vi "Configure Device.vi"(8 "error in":errorcluster, 11 "Vaisala Probe in":refnum<class "Vaisala.lvclass">) -> (0 "error out":errorcluster, 3 "Vaisala Probe out":refnum<class "Vaisala.lvclass">)   [LabVIEW 2015, in "Vaisala.lvclass"]
doc: "Configure the current instance of the Vaisala probe. In this case, we will get the correct address and then set the serial delayso that the probe responds in the correct amount of time. When configuration is done, make sure the session is closed."
uses:
  Vaisala.lvclass
  Instruments/Nicholas/Session/FPGA Serial Session.lvclass
  Reusable/Session APIs/File Access/Config Data/Config Data.lvclass
  Vaisala.lvclass/Vaisala.ctl
  Configurable Device/Configurable Device.lvclass/Configurable Device.ctl
  Reusable/Session APIs/File Access/Config Data/Config Data.lvclass/Config Data.ctl
  Reusable/Session APIs/Text Communication/Text Device Session.lvclass/Text Device Session.ctl
  Accessors/Read ID.vi
  Accessors/Read hSession.vi
  Configurable Device/Read Handle.vi
  Reusable/Session APIs/File Access/Config Data/Accessors/Read Ref.vi
  Reusable/Session APIs/Text Communication/Read hSysLog.vi
  <vilib>/Utility/config.llb/Read Key (I32).vi
  <userlib>/_Session Fwk/Session - Root.lvclass
  <vilib>/Utility/config.llb/NI_LVConfig.lvlib
  Reusable/Session APIs/Text Communication/Text Device Session.lvclass
  Reusable/Session APIs/Serial/Public/Get Data/Get String.vi
  Reusable/Session Log/System Log.lvclass
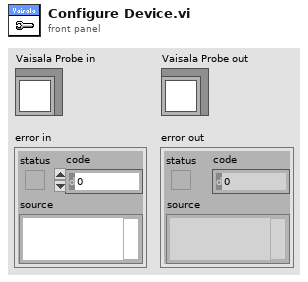
[diagram p1: front panel]
types:
  T1 = typedef "Session - Root.lvclass/Session Handle.ctl" = refnum<data-value>
  T2 = typedef "Config Data.lvclass/Config Session.ctl" = refnum<data-value>
  T3 = typedef "NI_LVConfig.lvlib/Config Data RefNum.ctl" = refnum<k1>
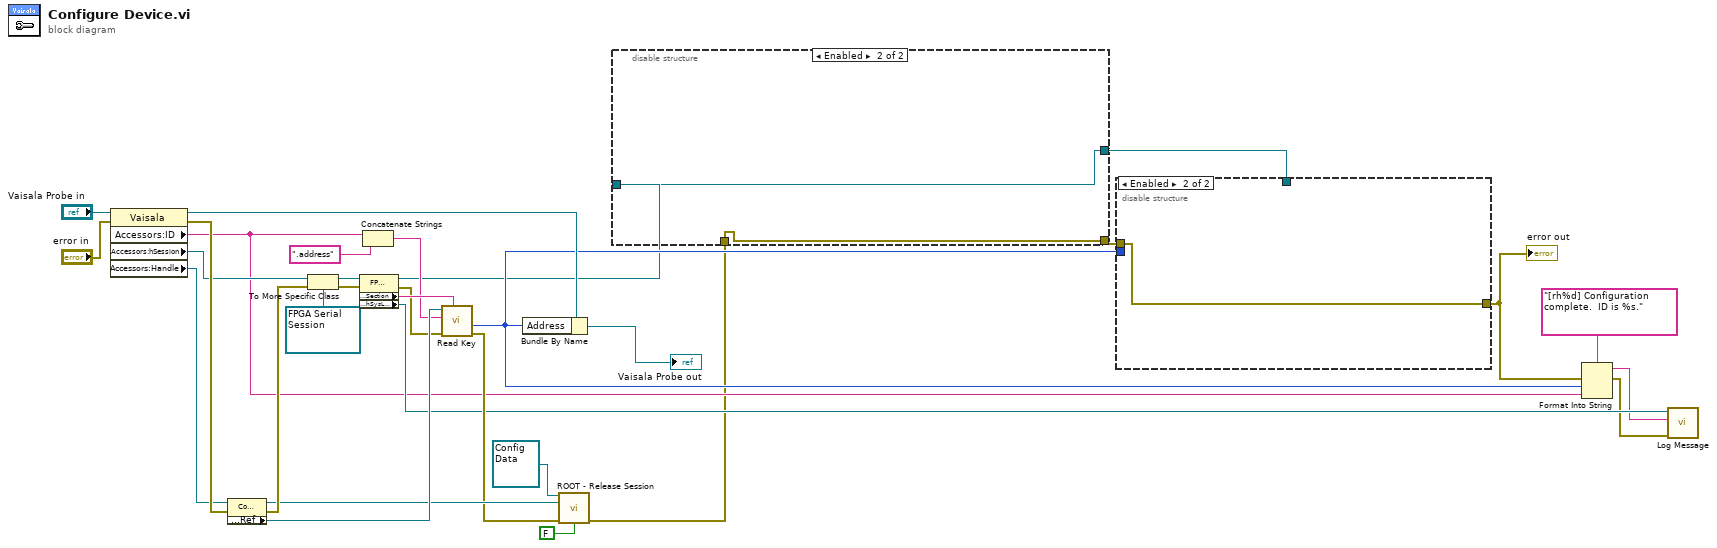
[diagram p0: block diagram]
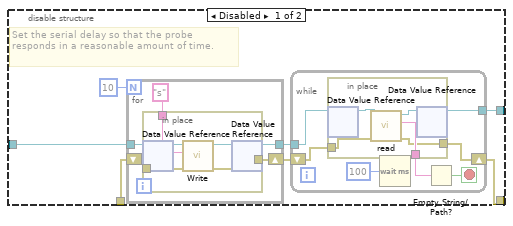
[diagram p2: hidden frame]
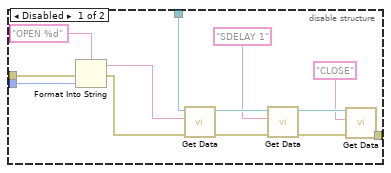
[diagram p3: hidden frame]
diagram:
  n1 = property class="Vaisala"(reference="Vaisala Probe in", error in="error in") -> (reference out=w24:refnum<class "Vaisala.lvclass">, error out=w21:errorcluster, "Accessors:ID"=w5:string, "Accessors:hSession"=w13:T1, "Accessors:Handle"=w12:T2)
  n2 = property class="Config Data"(reference=w12, error in=w21) -> (reference out=w17:T2, error out=w20:errorcluster, "Accessors:Ref"=w30:T3)
  n3 = To More Specific Class(target class=refnum<data-value> refnum ("hSession"), reference=w13, error in=w20) -> (specific class reference=w28:refnum<data-value>, error out=w19:errorcluster)
  n4 = property class="FPGA Serial Session"(reference=w28, error in=w19) -> (reference out=w4:refnum<data-value>, error out=w18:errorcluster, "Accessors:Section"=w27:string, "Accessors:hSysLog"=w11:T1)
  n5 = Concatenate Strings(w5, ".address" ("string")) -> (w25:string)
  n6 = call-poly <vilib>:"Read Key.vi"("section"=w27, "error in (no error)"=w18, "key"=w25, "refnum"=w30) -> ("error out"=w15:errorcluster, "value"=w6:i32)  [unwired: 4 in, 2 out]
  n7 = Bundle By Name(cluster=w24, "Address"=w6) -> (→"Vaisala Probe out":refnum<class "Vaisala.lvclass">)
  n8 = call <userlib>:"ROOT - Release Session.vi"("OBJ - Session in"=refnum<class "Config Data.lvclass"> refnum ("Config Data"), "Session Handle in"=w17, "error in (no error)"=w15, "force destroy? (F)"=FALSE) -> ("error out"=w2:errorcluster)  [unwired: 10 in, 1 out]
  n9 = disable-structure shown="Enabled" {
    disable-tunnel: w4 -> [w38 w61]
    disable-tunnel: [w35 w61] -> w3
    disable-tunnel: w2 -> [w34 w62]
    disable-tunnel: [w32 w62] -> w1
    frame Disabled {
      # "Set the serial delay so that the probe responds in a reasonable amount of time."
      n10 = for {
        N: 10 -> [_]
        tunnel: w38 -> [w55]
        tunnel: [w53] -> w36
        shift-right: [w51] -> w33
        shift-left: w34 -> [w52]
        n11 = in-place {
          in-place-border: "s" ("CMD") -> [w59]
          in-place-border: w52 -> [w57]
          in-place-border: [w56] -> w51
          n12 = in-place-dvr #1(w55) -> (w60:refnum<class "FPGA Serial Session.lvclass">)  [unwired: 1 out]
          n13 = call-dynamic "Write.vi"("error in"=w57, "Data In"=w59, "Text Session in"=w60) -> ("error out"=w56:errorcluster, "Text Session out"=w58:refnum<class "FPGA Serial Session.lvclass">)  [unwired: 7 in]
          n14 = in-place-dvr #1(w58) -> (w53:refnum<data-value>)  [unwired: 1 out]
        }
      }
      n15 = while {
        tunnel: w36 -> [w45]
        tunnel: [w41] -> w35
        shift-right: [w39] -> w32
        shift-left: w33 -> [w40]
        stop <- w43 stop-if-true
        n16 = in-place {
          in-place-border: [w48] -> w42
          in-place-border: w40 -> [w47]
          in-place-border: [w46] -> w39
          n17 = in-place-dvr #2(w45) -> (w50:refnum<class "FPGA Serial Session.lvclass">)  [unwired: 1 out]
          n18 = call-dynamic "read.vi"("error in"=w47, "Text Session in"=w50) -> ("error out"=w46:errorcluster, "Data Out"=w48:string, "Text Session out"=w49:refnum<class "FPGA Serial Session.lvclass">)  [unwired: 7 in]
          n19 = in-place-dvr #2(w49) -> (w41:refnum<data-value>)  [unwired: 1 out]
        }
        n20 = Wait (ms)(milliseconds to wait=u32 100) -> ()  [unwired: 1 out]
        n21 = Empty String/Path?(string/path=w42) -> (empty?=w43:bool)
      }
    }
    frame Enabled {
    }
  }
  n22 = disable-structure shown="Enabled" {
    disable-tunnel: w1 -> [w67 w76]
    disable-tunnel: [w65 w76] -> w8
    disable-tunnel: w6 -> [w64 _]
    disable-tunnel: w3 -> [w63 _]
    frame Disabled {
      n23 = Format Into String(format string="OPEN %d", error in=w67, w64) -> (resulting string=w74:string, error out=w66:errorcluster)  [unwired: 1 in]
      n24 = call-poly "Get Data.vi"("error in"=w66, "CMD"=w74, "handle in"=w63) -> ("error out"=w72:errorcluster, "handle out"=w73:T1)  [unwired: 6 in, 1 out]
      n25 = call-poly "Get Data.vi"("error in"=w72, "CMD"="SDELAY 1", "handle in"=w73) -> ("error out"=w69:errorcluster, "handle out"=w70:T1)  [unwired: 6 in, 1 out]
      n26 = call-poly "Get Data.vi"("error in"=w69, "CMD"="CLOSE", "handle in"=w70) -> ("error out"=w65:errorcluster)  [unwired: 6 in, 2 out]
    }
    frame Enabled {
    }
  }
  "error out" <- w8
  n27 = Format Into String(format string="[rh%d] Configuration complete.  ID is %s.", error in=w8, w6, w5) -> (resulting string=w7:string, error out=w9:errorcluster)  [unwired: 1 in]
  n28 = call "Log Message.vi"("error in"=w9, "MSG In"=w7, "session in"=w11) -> ()  [unwired: 7 in, 2 out]
